vi "SetAtt.vi"(2 "Arm Trigs?":bool, 4 "Attenuation":u8(slide) scale=0.0..63.0, 5 "Port Address":u32=888 format="%.0x") -> ()   [LabVIEW 2022 SP3]
uses:
  <vilib>/DAQmx/write.llb/DAQmx Write (Digital 1D U8 NChan 1Samp).vi
  <vilib>/DAQmx/miscellaneous.llb/DAQmx Fill In Error Info.vi
  <instrlib>/vi.lib/Platform/portaccess.llb/Out Port8.vi
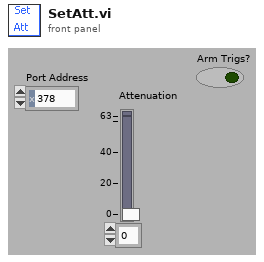
[diagram p1: front panel]
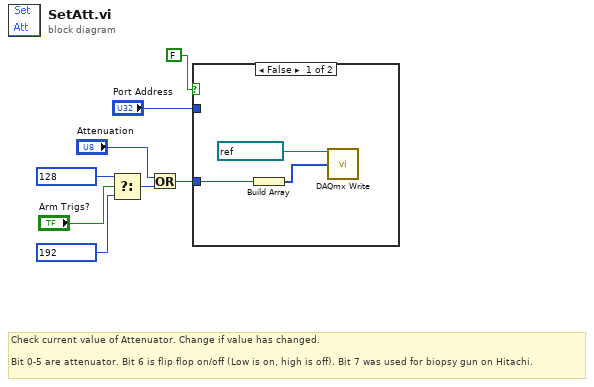
[diagram p0: block diagram]
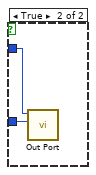
[diagram p2: hidden frame]
diagram:
  # "Check current value of Attenuator. Change if value has changed.\n\nBit 0-5 are attenuator. Bit 6 is flip flop on/off (Low is on, high is off). Bit 7 was used for biopsy gun on Hitachi."
  n1 = Select(t=u8 128, s="Arm Trigs?", f=u8 192) -> (s? t:f=w3:u8)
  n2 = Or(x="Attenuation", y=w3) -> (x .or. y?=w2:u8)
  n3 = case shown="False" FALSE ("Case Constant\n(See Context Help)") {
    tunnel: "Port Address" -> [_ w13]
    tunnel: w2 -> [w10 w12]
    frame False {
      n4 = Build Array(w10) -> (w9:u8[])
      n5 = call-poly <vilib>:"DAQmx Write.vi"("task/channels in"=refnum<k21> "Hitachi", "data"=w9) -> ()  [unwired: 11 in, 3 out]
    }
    frame True {
      n6 = call-poly <instrlib>:"Out Port.vi"("write value"=w12, "address"=w13) -> ()  [unwired: 1 in, 7 out]
    }
  }
